vi "Module - DAQmx AI.vi"(8 "Error In":errorcluster) -> (0 "Error Out":errorcluster)   [LabVIEW 2020]
uses:
  Control/State - DAQmx AI.ctl
  Control/State - eFGV.ctl
  Control/FGV State.ctl
  Control/Section Config RT.ctl
  <vilib>/DAQmx/read.llb/DAQmx Read (Analog 1D Wfm NChan NSamp).vi
  <vilib>/DAQmx/create/channels.llb/DAQmx Create Channel (AI-Bridge).vi
  <vilib>/DAQmx/configure/timing.llb/DAQmx Timing (Sample Clock).vi
  <vilib>/DAQmx/miscellaneous.llb/DAQmx Fill In Error Info.vi
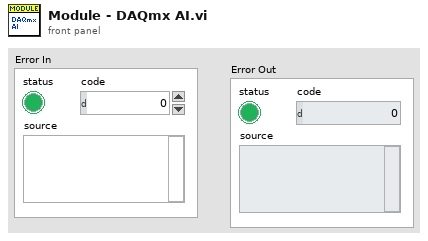
[diagram p1: front panel]
types:
  T1 = cluster{"T_Out":i32, "Physical Channel":tag[], "DAQmx Task Ref.":refnum<k21>, "IO Tags":string[], "Channel Created?":bool, "Sampling rate":i32, "Stop Main RT":bool, "sampleInterval":u32, "AI Raw Data":waveform(dbl)[], "Event Ref":refnum<event-registration>, "I/Os":tag[]}
  T2 = typedef "State - DAQmx AI.ctl" = enum16{"Init", "Register Event", "Read IO Setting", "Create Channel", "Timing Setting", "Register DAQmx Event", "Start Task", "Read Cal Config", "Idle", "DAQmx Read", "Scale", "Send eFGV", "Stop Task", "Unregister Event", "Close"}
  T3 = typedef "State - eFGV.ctl" = enum16{"Init", "Read", "Write", "Exit"}
  T4 = typedef "FGV State.ctl" = enum16{"Write", "Read"}
  T5 = cluster{"bridge configuration":i32, "voltage excitation source":i32, "voltage excitation value":dbl, "nominal bridge resistance":dbl}
  T6 = typedef "Section Config RT.ctl" = enum16{"Mod1/AI0", "Mod1/AI1", "Mod1/AI2", "Mod1/AI3", "Network Stream", "Acquisition Setting"}
  T7 = typedef "Modules Info.ctl" = cluster{"Product Name":string, "Product Type ":string, "I/Os":tag[]}
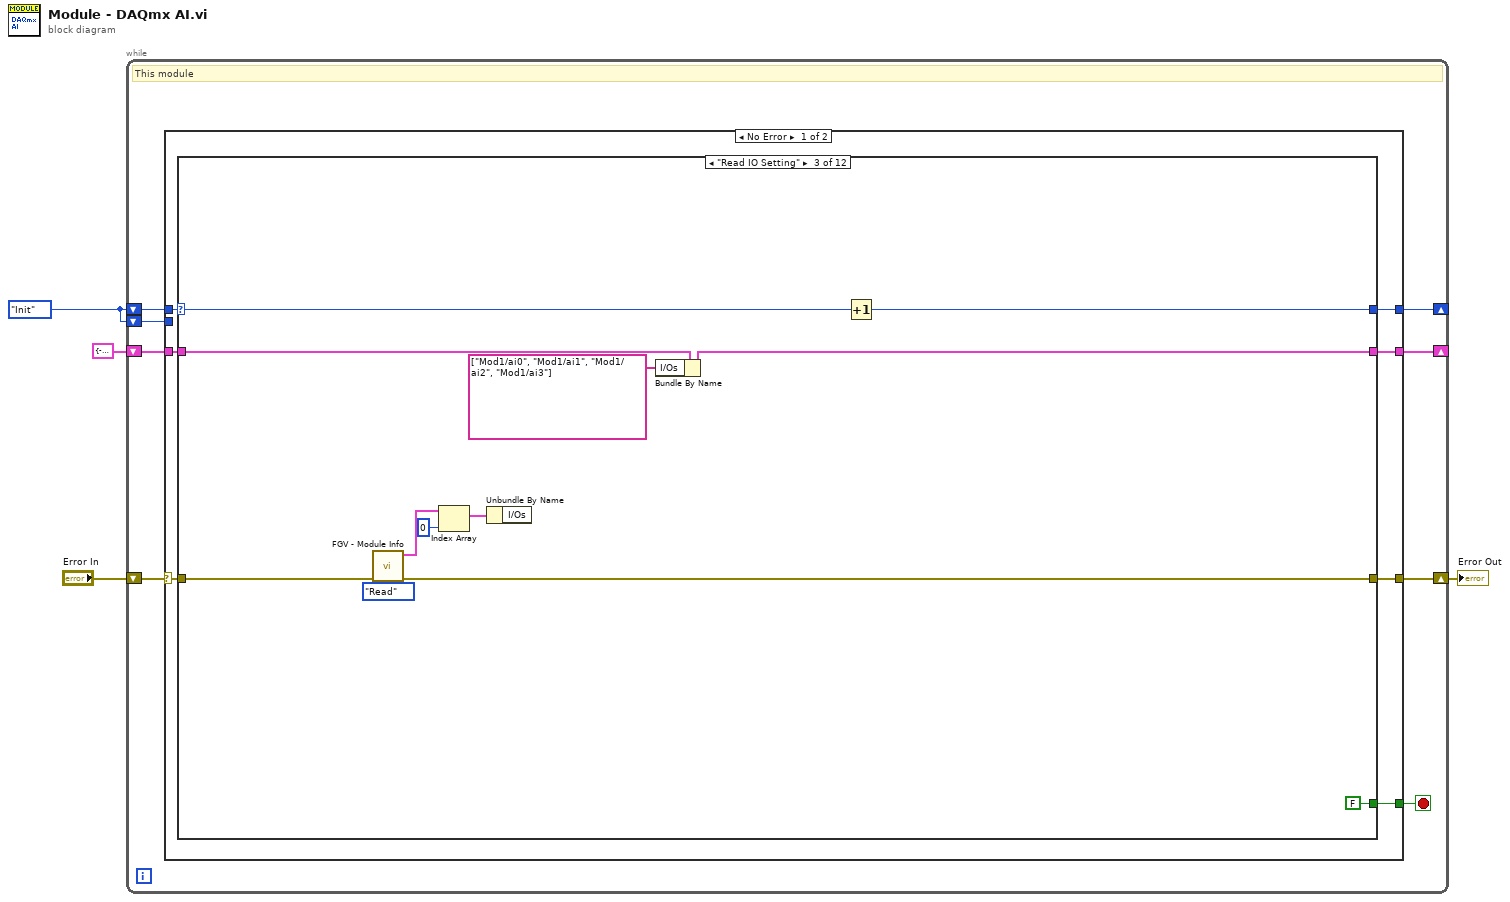
[diagram p0: block diagram]
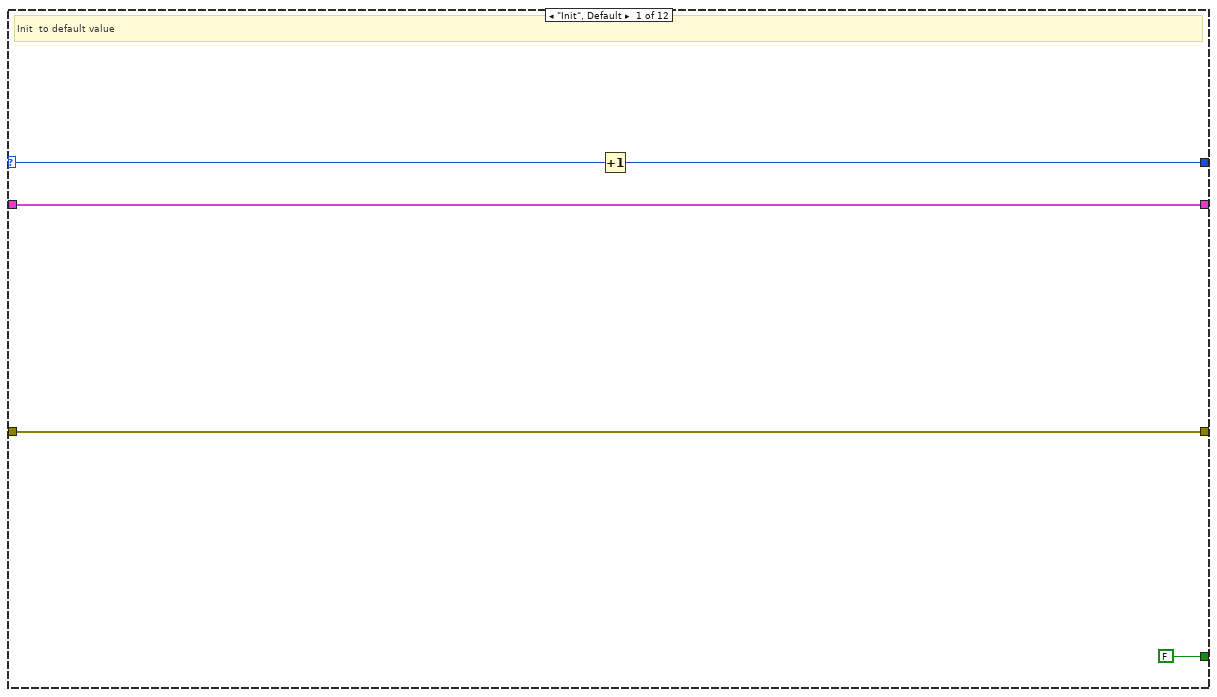
[diagram p2: hidden frame]
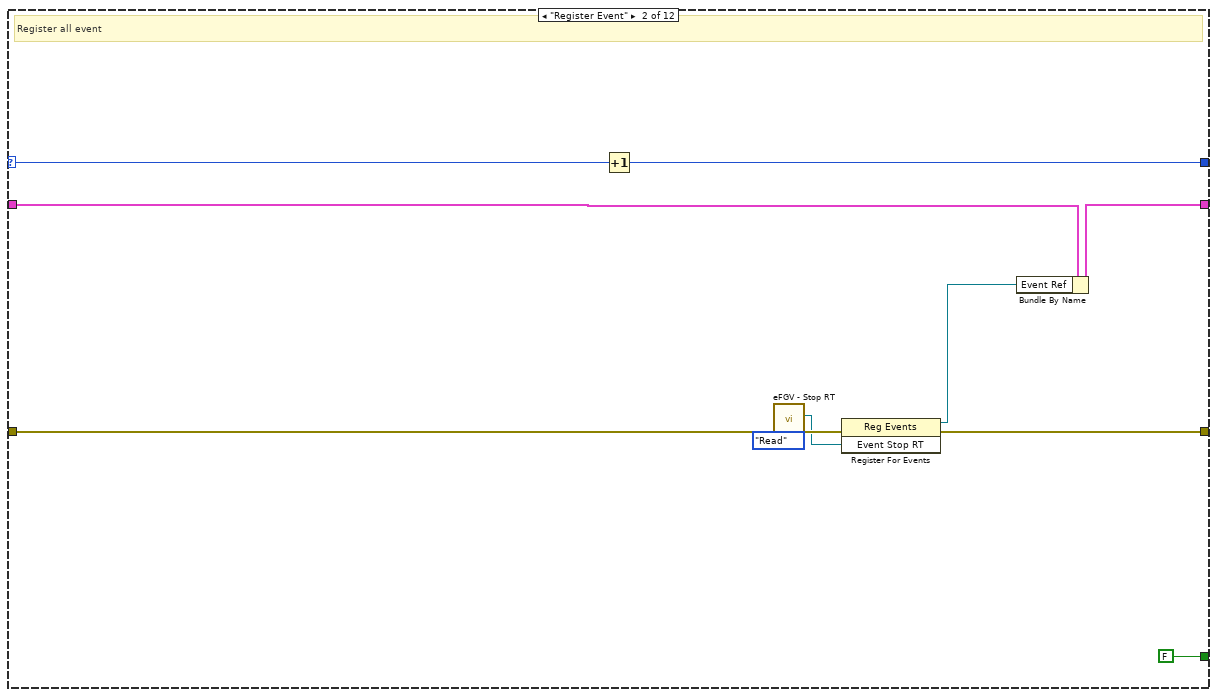
[diagram p3: hidden frame]
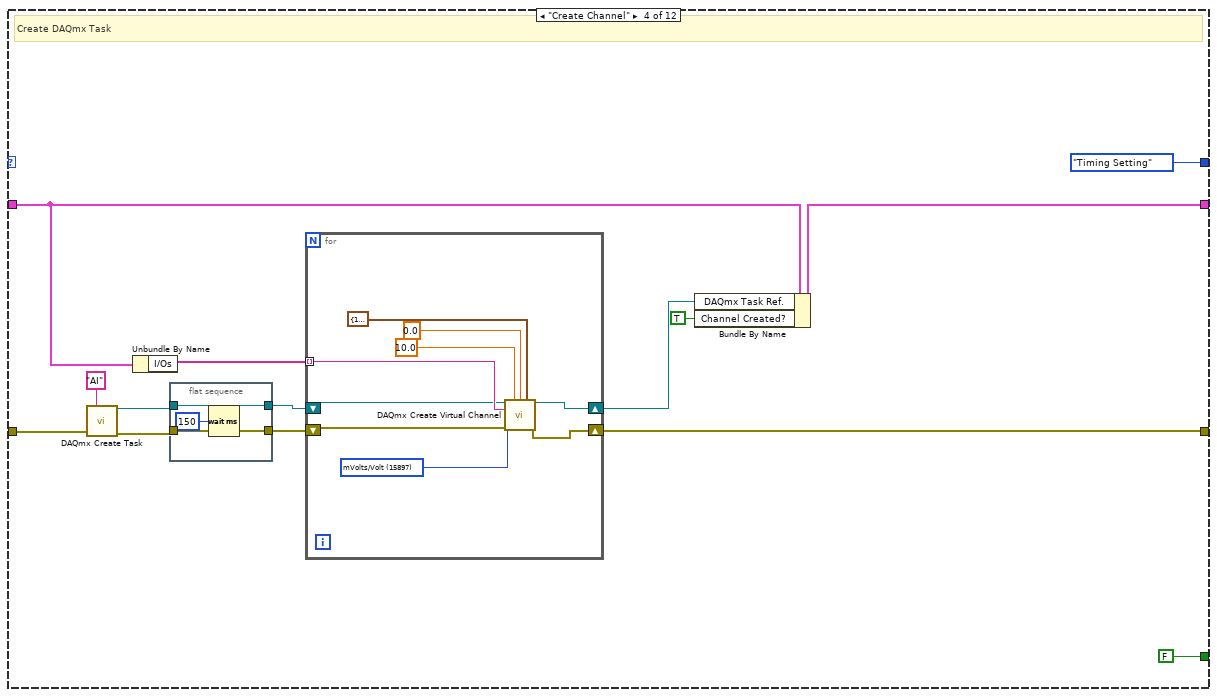
[diagram p4: hidden frame]
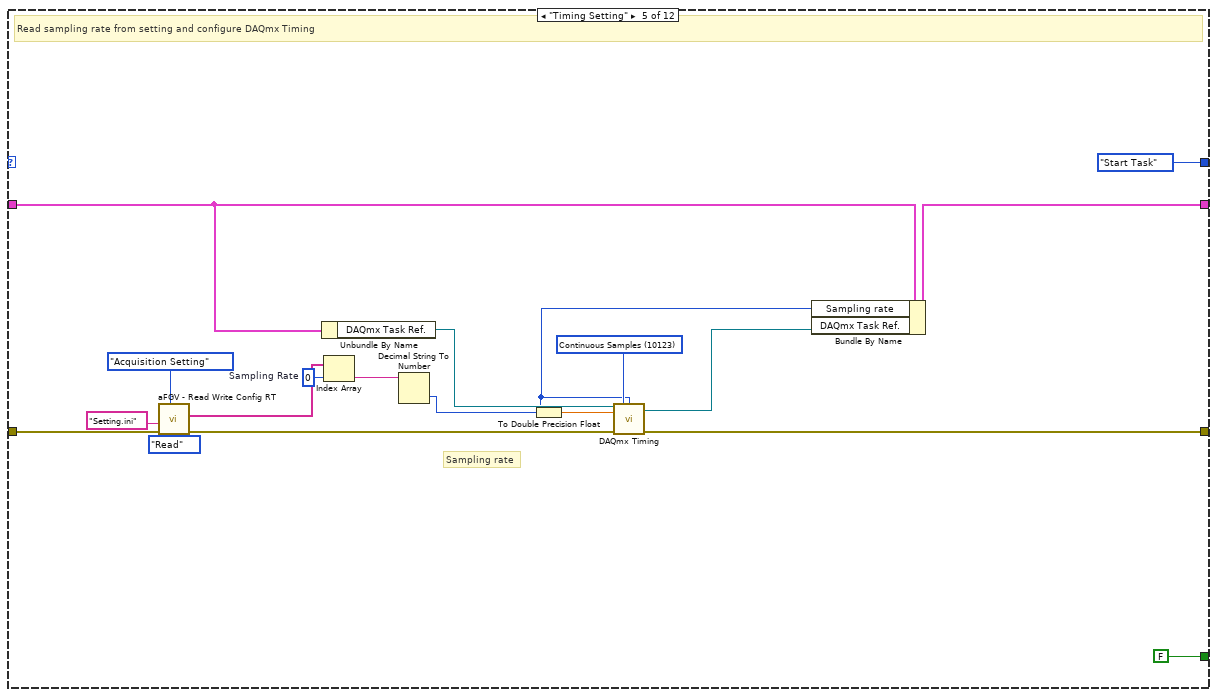
[diagram p5: hidden frame]
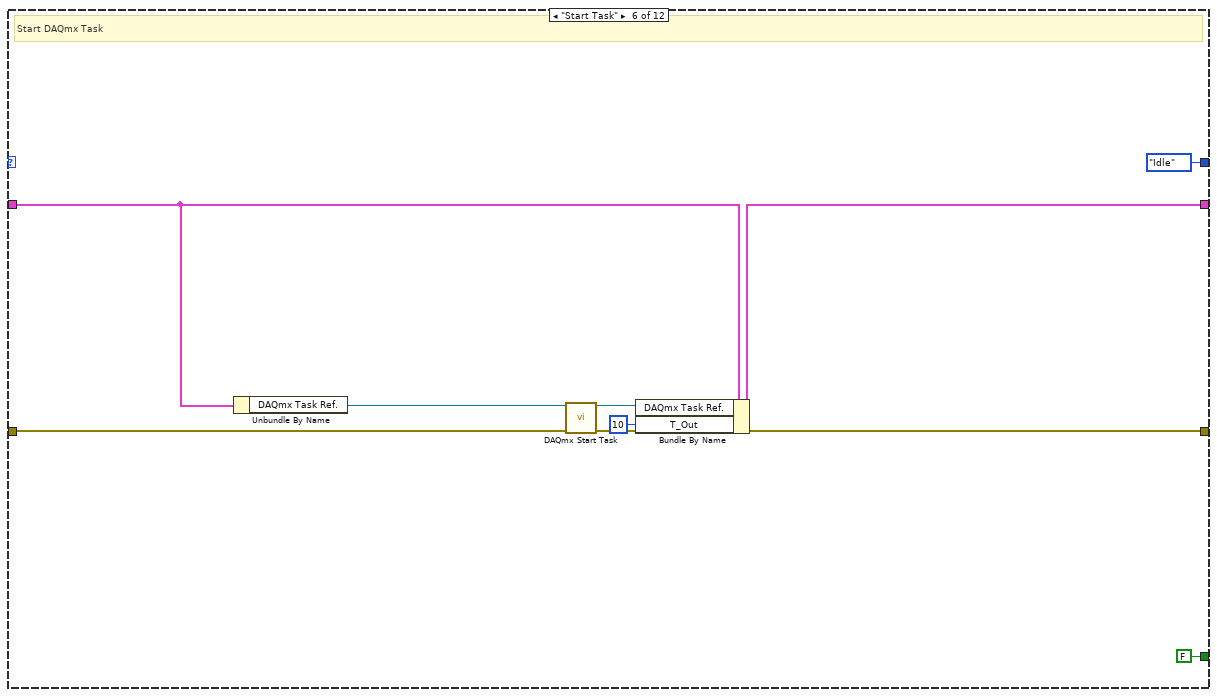
[diagram p6: hidden frame]
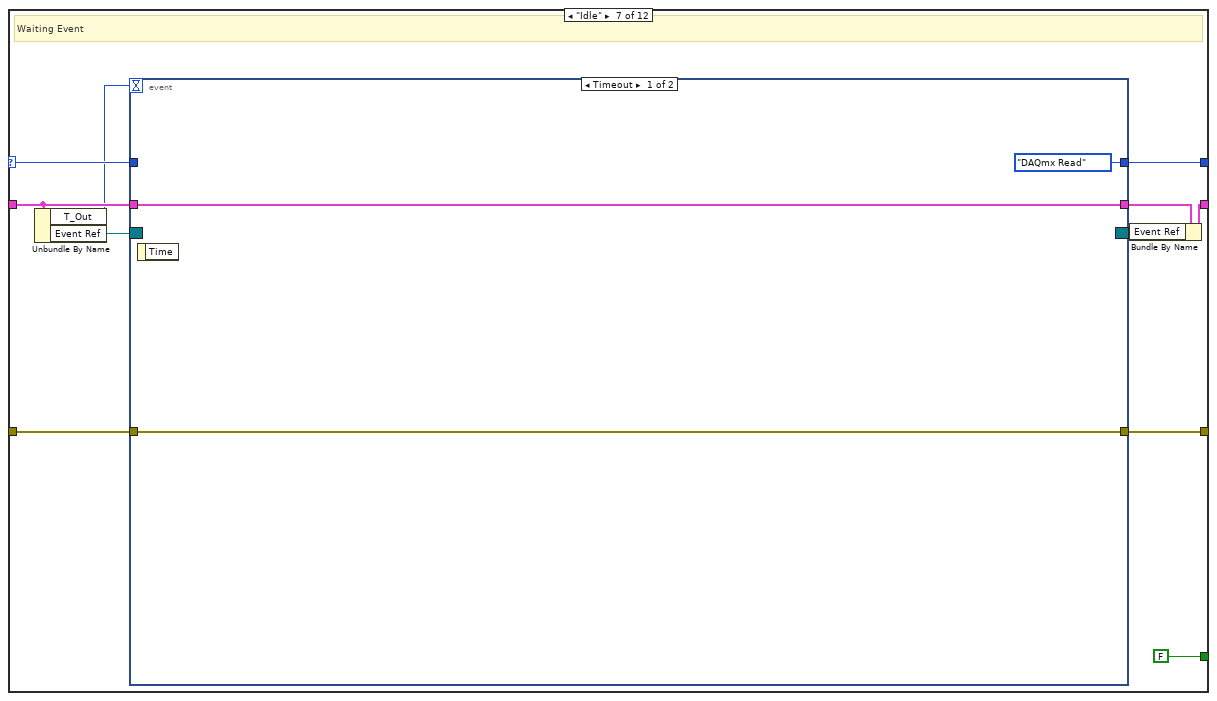
[diagram p7: hidden frame]
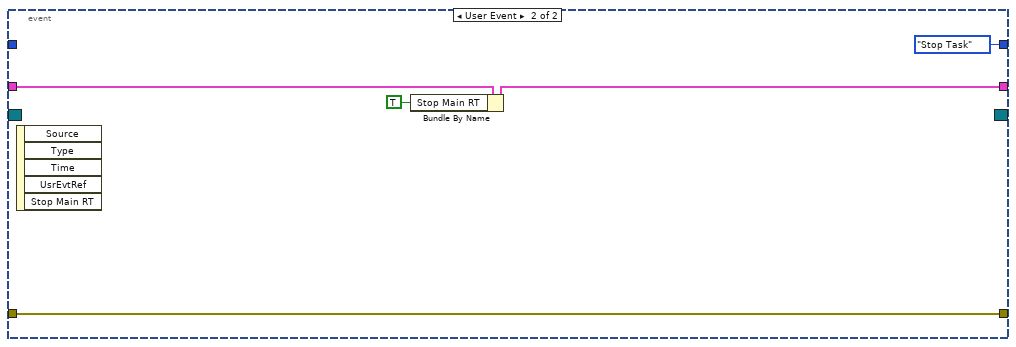
[diagram p8: hidden frame]
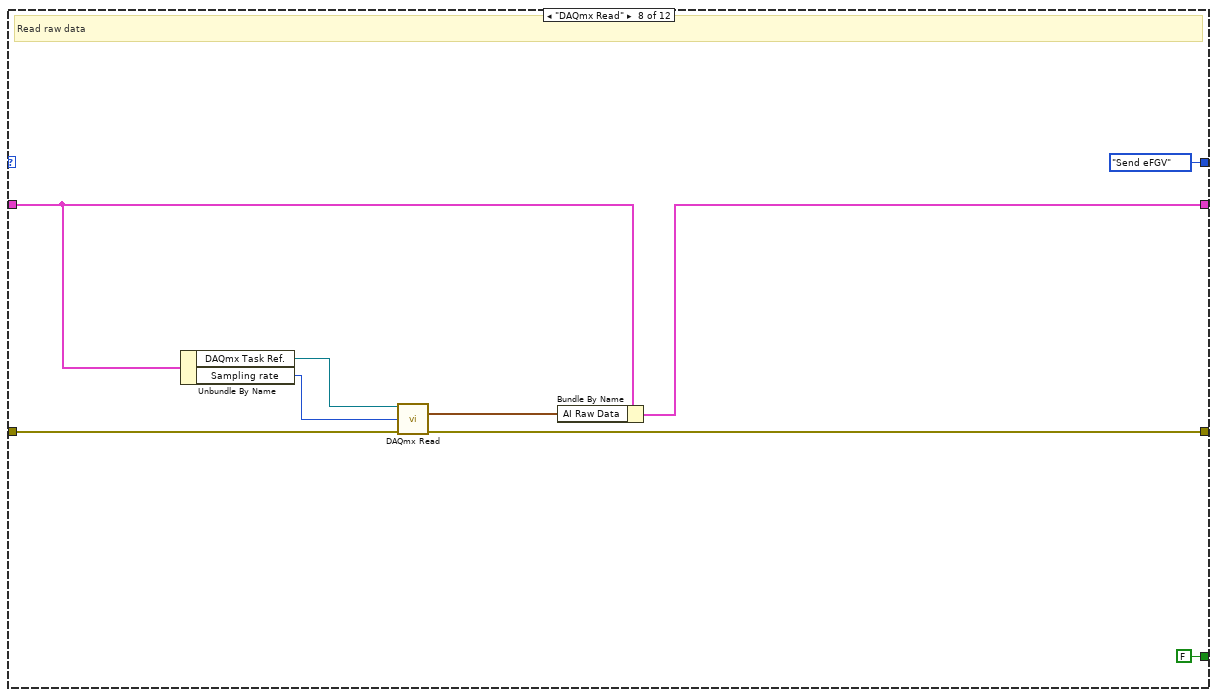
[diagram p9: hidden frame]
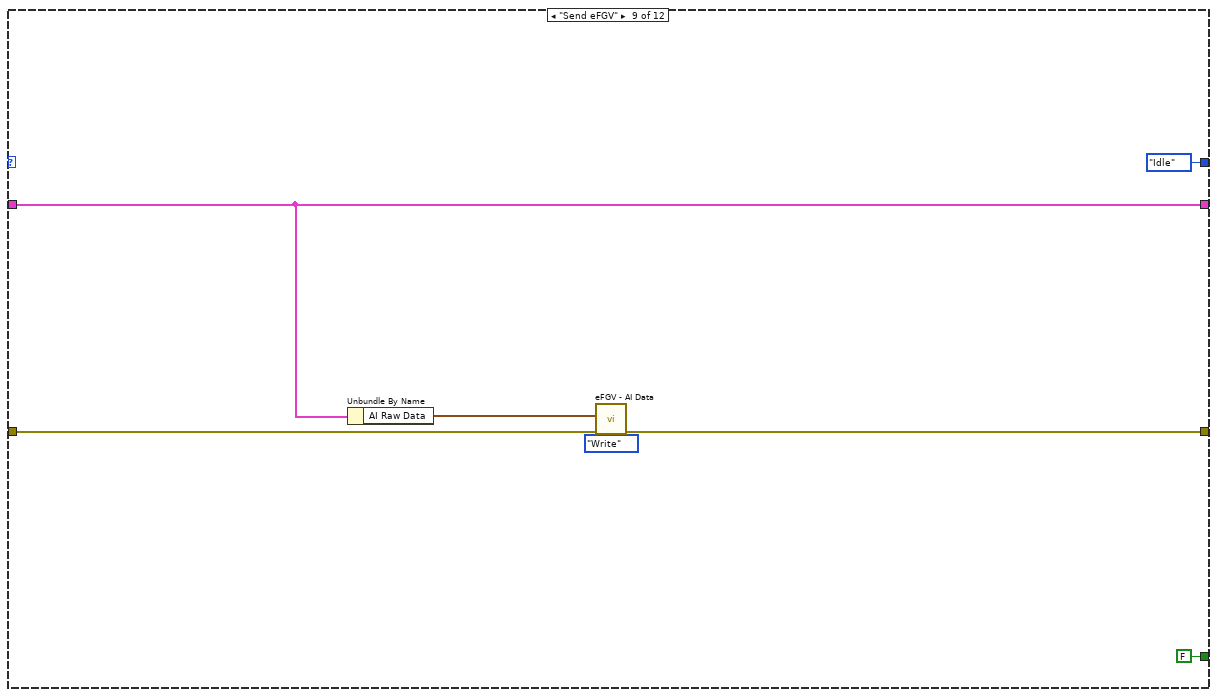
[diagram p10: hidden frame]
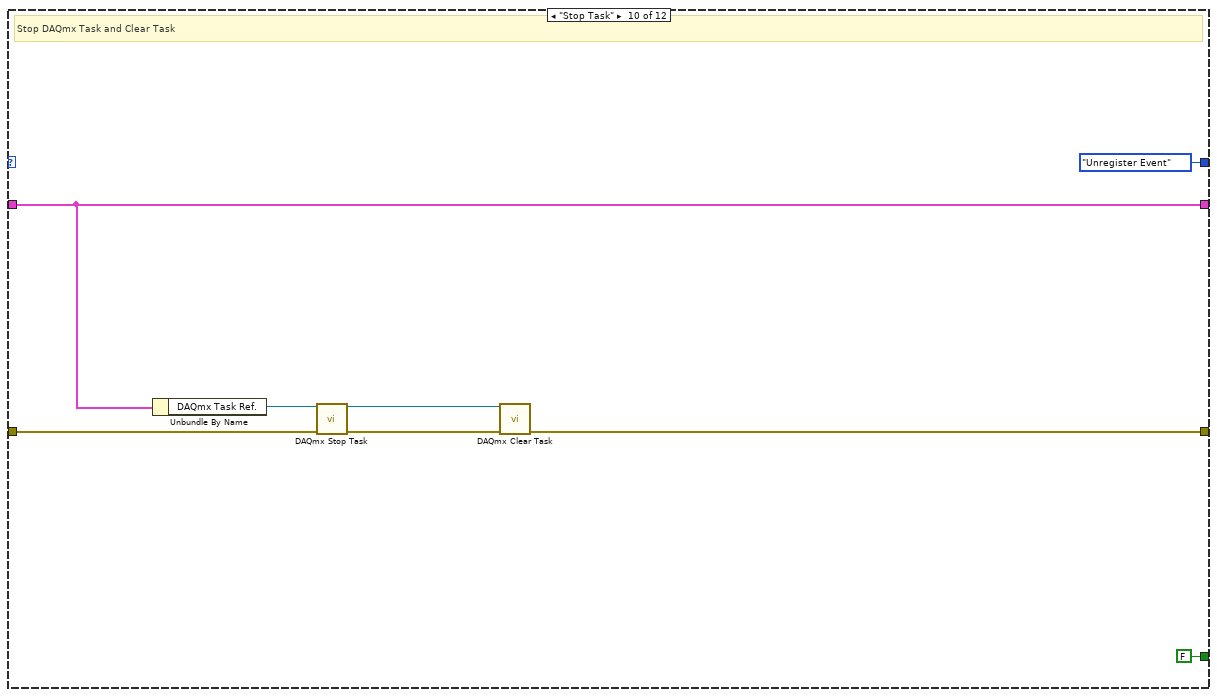
[diagram p11: hidden frame]
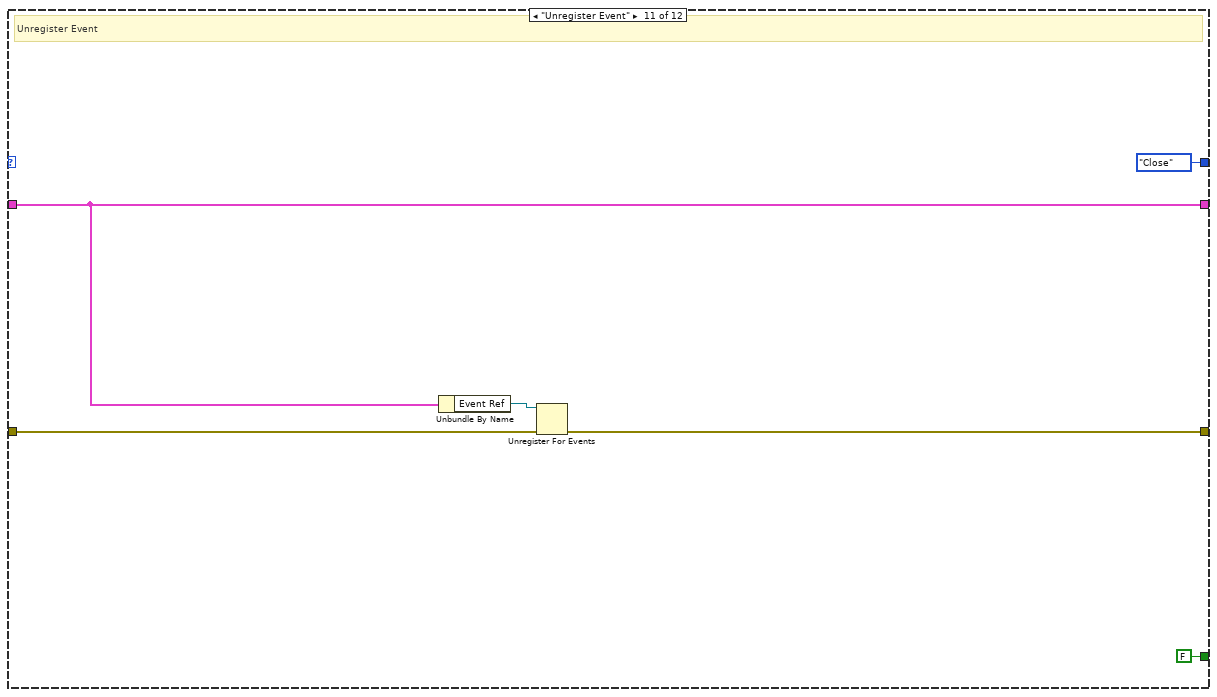
[diagram p12: hidden frame]
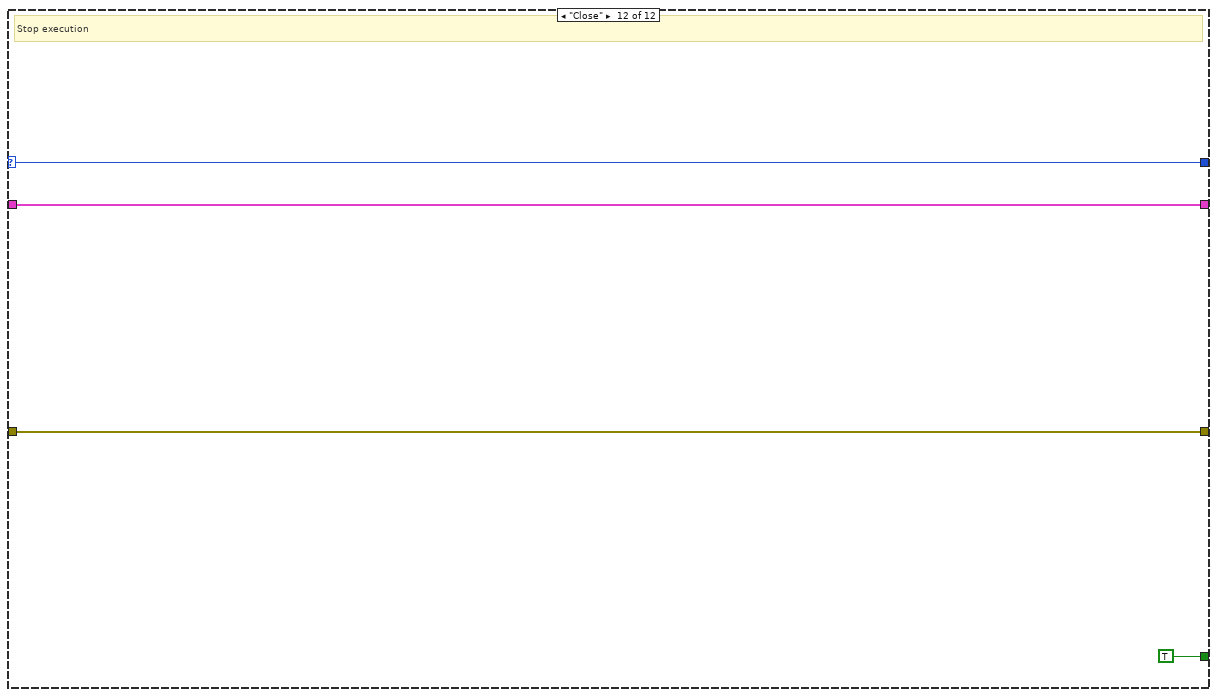
[diagram p13: hidden frame]
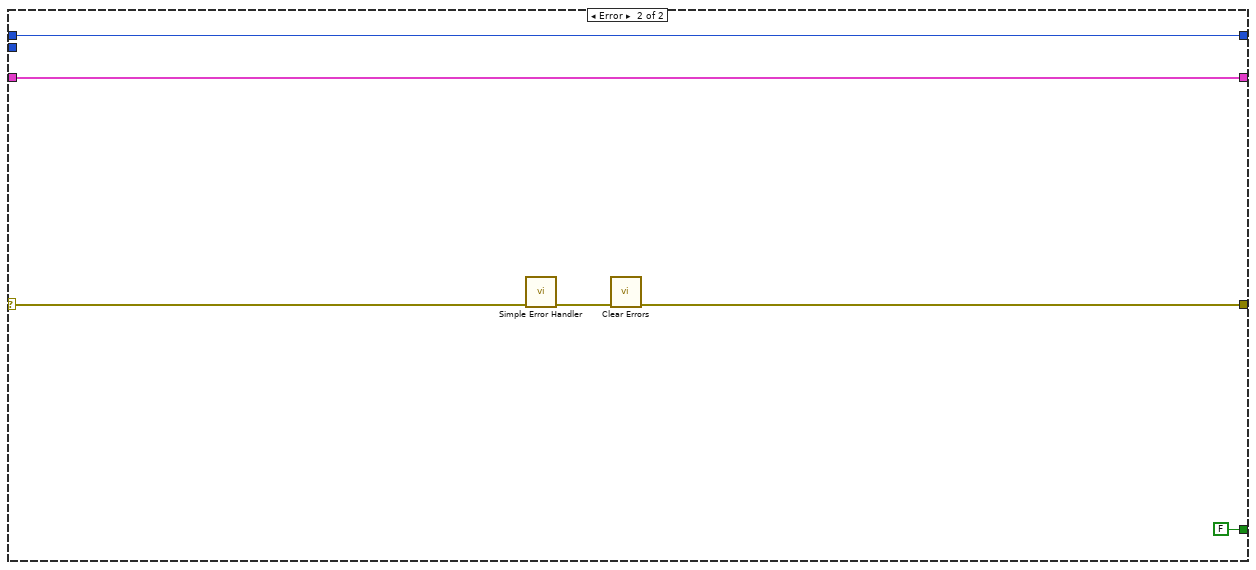
[diagram p14: hidden frame]
diagram:
  w4 = State_-_DAQmx_AI."Init"
  n1 = while {
    shift-right: [w8] -> _
    shift-left: w4 -> [w10]
    shift-right: [w11] -> w2
    shift-left: "Error In" -> [w12]
    shift-right: [w6] -> _
    shift-left: T1 {"T_Out"=-1, "Physical Channel"=[], "DAQmx Task Ref."="", "IO Tags"=[], "Channel Created?"=FALSE, "Sampling rate"=0, "Stop Main RT"=FALSE, "sampleInterval"=0, "AI Raw Data"=[], "Event Ref"=refnum, "I/Os"=[]} -> [w7]
    shift-left: w4 -> [w5]
    stop <- w9 stop-if-true
    # "This module"
    n2 = case shown="No Error" w12 {
      selector: w12 -> [w18 w156]
      tunnel: w10 -> [w17 w158]
      tunnel: [w19 w155] -> w11
      tunnel: [w16 FALSE] -> w9
      tunnel: [w15 w158] -> w8
      tunnel: w7 -> [w14 w157]
      tunnel: [w13 w157] -> w6
      tunnel: w5 -> [_ _]
      frame No Error {
        n3 = case shown="\"Read IO Setting\"" w17 {
          selector: w17 -> [w21 w32 w38 _ _ _ w106 _ _ _ _ w151]
          tunnel: [w24 w35 w43 w51 w90 w97 w111 w123 w132 w140 w148 w153] -> w19
          tunnel: w18 -> [w24 w27 w45 w59 w89 w100 w110 w124 w133 w137 w149 w153]
          tunnel: [FALSE FALSE FALSE FALSE FALSE FALSE FALSE FALSE FALSE FALSE FALSE TRUE] -> w16
          tunnel: [w20 w30 w37 State_-_DAQmx_AI."Timing Setting" State_-_DAQmx_AI."Start Task" State_-_DAQmx_AI."Idle" w108 State_-_DAQmx_AI."Send eFGV" State_-_DAQmx_AI."Idle" State_-_DAQmx_AI."Unregister Event" State_-_DAQmx_AI."Close" w151] -> w15
          tunnel: w14 -> [w23 w29 w47 w49 w82 w96 w105 w128 w130 w143 w147 w152]
          tunnel: [w23 w28 w39 w57 w80 w94 w103 w125 w130 w143 w147 w152] -> w13
          frame "Init", Default {
            # "Init  to default value"
            n4 = Increment(x=w21) -> (x+1=w20:T2)
          }
          frame "Register Event" {
            # "Register all event"
            n5 = Increment(x=w32) -> (x+1=w30:T2)
            n6 = call "eFGV - Stop RT.vi"("State"=State_-_eFGV."Read", "Error In"=w27) -> ("Error Out"=w34:errorcluster, "Event Stop RT"=w31:refnum<user-event>)  [unwired: 7 in, 1 out]
            n7 = register-events(error in=w34, w31) -> (reference out=w25:refnum<event-registration>, error out=w35:errorcluster)  [unwired: 1 in]
            n8 = Bundle By Name(cluster=w29, "Event Ref"=w25) -> (w28:T1)
          }
          frame "Read IO Setting" {
            n9 = call "FGV - Module Info.vi"("FGV State"=FGV_State."Read", "Error In"=w45) -> ("Error Out"=w43:errorcluster, "Module Info"=w42:T7[])  [unwired: 8 in]
            n10 = Index Array(array=w42, index=0) -> (element=w41:T7)
            n11 = Unbundle By Name(w41) -> ()  [unwired: 1 out]
            n12 = Bundle By Name(cluster=w47, "I/Os"=tag[] ["Mod1/ai0", "Mod1/ai1", "Mod1/ai2", "Mod1/ai3"]) -> (w39:T1)
            n13 = Increment(x=w38) -> (x+1=w37:T2)
          }
          frame "Create Channel" {
            # "Create DAQmx Task"
            n14 = call <vilib>:"DAQmx Create Task.vi"("new task name"="AI", "error in"=w59) -> ("task out"=w52:refnum<k21>, "error out"=w53:errorcluster)  [unwired: 12 in]
            n15 = Unbundle By Name(w49) -> ("I/Os"=w48:tag[])
            n16 = flat-sequence {
              tunnel: w53 -> [w73]
              tunnel: [w73] -> w55
              tunnel: w52 -> [w72]
              tunnel: [w72] -> w54
              frame #0 {
                n17 = Wait (ms)(milliseconds to wait=u32 150) -> ()  [unwired: 1 out]
              }
            }
            n18 = for {
              tunnel: w48 -> [w70] mode=indexing
              shift-right: [w63] -> w51
              shift-left: w55 -> [w69]
              shift-right: [w62] -> w50
              shift-left: w54 -> [w68]
              w65 = 15897 items=["Volts/Volt"=15896, "mVolts/Volt"=15897, "From Custom Scale"=10065] ("units")
              n19 = call-poly <vilib>:"DAQmx Create Virtual Channel.vi"("task in"=w68, "maximum value"=10.0, "minimum value"=0.0, "bridge information"=T5 {"bridge configuration"=10182, "voltage excitation source"=10200, "voltage excitation value"=10.0, "nominal bridge resistance"=350.0}, "physical channels"=w70, "units"=w65, "error in"=w69) -> ("task out"=w62:refnum<k21>, "error out"=w63:errorcluster)  [unwired: 7 in]
            }
            n20 = Bundle By Name(cluster=w49, "DAQmx Task Ref."=w50, "Channel Created?"=TRUE) -> (w57:T1)
          }
          frame "Timing Setting" {
            w85 = 0  # Sampling Rate
            w78 = 10123 items=["Finite Samples"=10178, "Continuous Samples"=10123, "Hardware Timed Single Point"=12522] ("sample mode")
            # "Sampling rate"
            # "Read sampling rate from setting and configure DAQmx Timing"
            n21 = call "aFGV - Read Write Config RT.vi"("State"=enum16{"Read", "Write", "Delete"}."Read", "Section"=Section_Config_RT."Acquisition Setting", "Error In"=w89, "File name"="Setting.ini" ("Filename")) -> ("Error Out"=w88:errorcluster, "Data out"=w86:string[])  [unwired: 5 in, 1 out]
            n22 = Unbundle By Name(w82) -> ("DAQmx Task Ref."=w81:refnum<k21>)
            n23 = Index Array(array=w86, index=w85) -> (element=w84:string)
            n24 = Decimal String To Number(string=w84) -> (number=w75:i32)  [unwired: 2 in, 1 out]
            n25 = To Double Precision Float(number=w75) -> (double precision float=w76:dbl)
            n26 = call-poly <vilib>:"DAQmx Timing.vi"("task/channels in"=w81, "sample mode"=w78, "samples per channel"=w75, "rate"=w76, "error in"=w88) -> ("task out"=w79:refnum<k21>, "error out"=w90:errorcluster)  [unwired: 9 in]
            n27 = Bundle By Name(cluster=w82, "Sampling rate"=w75, "DAQmx Task Ref."=w79) -> (w80:T1)
          }
          frame "Start Task" {
            # "Start DAQmx Task"
            n28 = Unbundle By Name(w96) -> ("DAQmx Task Ref."=w95:refnum<k21>)
            n29 = call <vilib>:"DAQmx Start Task.vi"("task/channels in"=w95, "error in"=w100) -> ("task out"=w93:refnum<k21>, "error out"=w97:errorcluster)  [unwired: 12 in]
            n30 = Bundle By Name(cluster=w96, "DAQmx Task Ref."=w93, "T_Out"=10) -> (w94:T1)
          }
          frame "Idle" {
            # "Waiting Event"
            n31 = Unbundle By Name(w105) -> ("T_Out"=w101:i32, "Event Ref"=w104:refnum<event-registration>)
            n32 = event shown="[0] Timeout" {
              selector: w104 -> [_ _]
              dyn-events: [_ _] -> w102
              timeout: w101 -> [_ _]
              tunnel: [w114 w119] -> w111
              tunnel: w110 -> [w114 w119]
              tunnel: [State_-_DAQmx_AI."DAQmx Read" State_-_DAQmx_AI."Stop Task"] -> w108
              tunnel: [w113 w116] -> w107
              tunnel: w105 -> [w113 w118]
              tunnel: w106 -> [_ _]
              event Timeout {
                n33 = event-data() -> ()  [unwired: 1 in, 1 out]
              }
              event User Event {
                n34 = event-data() -> ()  [unwired: 1 in, 5 out]
                n35 = Bundle By Name(cluster=w118, "Stop Main RT"=TRUE) -> (w116:T1)
              }
            }
            n36 = Bundle By Name(cluster=w107, "Event Ref"=w102) -> (w103:T1)
          }
          frame "DAQmx Read" {
            # "Read raw data"
            n37 = Unbundle By Name(w128) -> ("DAQmx Task Ref."=w122:refnum<k21>, "Sampling rate"=w120:i32)
            n38 = call-poly <vilib>:"DAQmx Read.vi"("task/channels in"=w122, "number of samples per channel"=w120, "error in"=w124) -> ("data"=w121:waveform(dbl)[], "error out"=w123:errorcluster)  [unwired: 10 in, 1 out]
            n39 = Bundle By Name(cluster=w128, "AI Raw Data"=w121) -> (w125:T1)
          }
          frame "Send eFGV" {
            n40 = Unbundle By Name(w130) -> ("AI Raw Data"=w129:waveform(dbl)[])
            n41 = call "eFGV - AI Data.vi"("States"=State_-_eFGV."Write", "Error In"=w133, "AI Agg"=w129) -> ("Error Out"=w132:errorcluster)  [unwired: 7 in, 1 out]
          }
          frame "Stop Task" {
            # "Stop DAQmx Task and Clear Task"
            n42 = Unbundle By Name(w143) -> ("DAQmx Task Ref."=w139:refnum<k21>)
            n43 = call <vilib>:"DAQmx Stop Task.vi"("task/channels in"=w139, "error in"=w137) -> ("task out"=w136:refnum<k21>, "error out"=w138:errorcluster)  [unwired: 12 in]
            n44 = call <vilib>:"DAQmx Clear Task.vi"("task in"=w136, "error in"=w138) -> ("error out"=w140:errorcluster)  [unwired: 13 in]
          }
          frame "Unregister Event" {
            # "Unregister Event"
            n45 = Unbundle By Name(w147) -> ("Event Ref"=w146:refnum<event-registration>)
            n46 = Unregister For Events(event registration refnum=w146, error in=w149) -> (error out=w148:errorcluster)
          }
          frame "Close" {
            # "Stop execution"
          }
        }
      }
      frame Error {
        n47 = call <vilib>:"Simple Error Handler.vi"("error in (no error)"=w156) -> ("error out"=w154:errorcluster)  [unwired: 4 in, 4 out]
        n48 = call <vilib>:"Clear Errors.vi"("error in (no error)"=w154) -> ("error out"=w155:errorcluster)  [unwired: 5 in, 1 out]
      }
    }
  }
  "Error Out" <- w2
